vi "run.vi"(8 "error in (no error)":errorcluster, 11 "DL090130ExperimentController in":refnum<class "ExperimentControllerDL090130Interval.lvclass">=refnum) -> (0 "error out":errorcluster, 3 "DL090130ExperimentController out":refnum<class "ExperimentControllerDL090130Interval.lvclass">)   [LabVIEW 2010, in "ExperimentControllerDL090130Interval.lvclass"]
uses:
  ExperimentControllerDL090130Interval.lvclass
  common/classes/SpaceVector/SpaceVector/SpaceVector.lvclass
  Sweep/GenericSweep/GenericSweep/GenericSweep.lvclass
  schedule_entry_cluster.ctl
  internal_trigger_enum.ctl
  main/labview_source/controls/undock_button.ctl
  ExperimentControllerDL090130Interval.lvclass/ExperimentControllerDL090130Interval.ctl
  GenericExperimentController/GenericExperimentController/GenericExperimentController.lvclass
  common/classes/GenericToplevelComponent/GenericToplevelComponent/trigger_type_enum.ctl
  GenericExperimentController/GenericExperimentController/trigger_enum.ctl
  common/classes/ErrorController/ErrorController/class_data.vi
  common/classes/ErrorController/ErrorController/ErrorController.lvclass
panel:
  in  "button:undock":T1
  in  "Tab Control":enum32{"User", "Debug", "About"}(tab)
  in  "number of sweeps":i32=1
  in  "sweep period":dbl[unit]
  in  "current sweep":i32
  in  "configure sweep button":bool
  out "event str time-out":i32
  out "stop?":bool
  in  "scheduled triggers":T2[](array[typedef])
  out "any triggers scheduled?":bool
  out "time-out for next sweep":i32
  out "last time-out: trigger due?":bool
  out "last trigger":T2
  out "last trigger time":timestamp
  out "evnt loop error":errorcluster
  out "last trigger":T3
  out "event handling loop counter":i32=343
  # "Sweep period:  duration from the beginning of one sweep to the beginning of the next sweep.\nImportant: The sweep period has to be longer than the actual duration of the sweep (including possible saving)."
  # "ExperimentControllerDL090130Interval\n\nImplemented by:\nDominik Langer, University of Zurich, Switzerland"
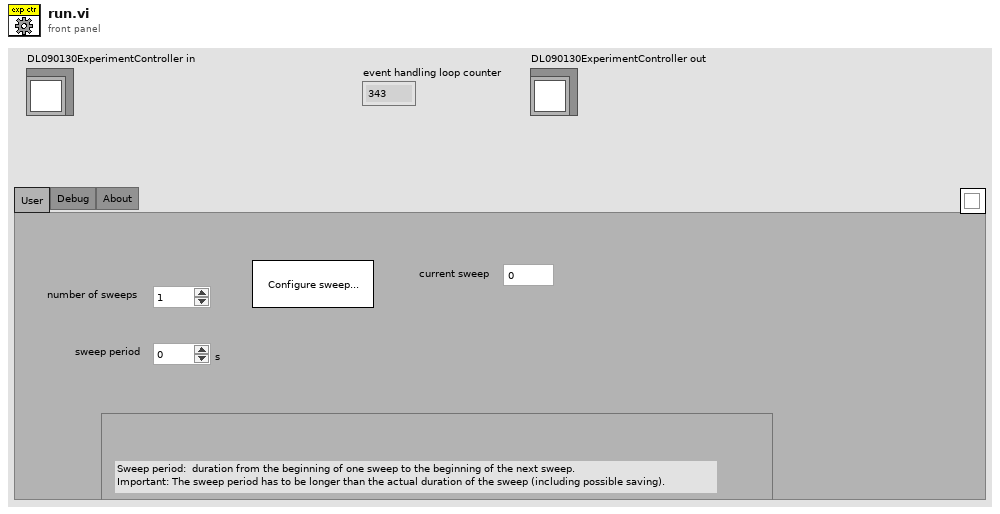
[diagram p1: front panel]
types:
  T1 = typedef "undock_button.ctl" = bool
  T2 = typedef "ExperimentControllerDL090130Interval.lvclass/schedule_entry_cluster.ctl" = cluster{"time":timestamp, "trigger":T3}
  T3 = typedef "ExperimentControllerDL090130Interval.lvclass/internal_trigger_enum.ctl" = enum16{"NULL", "initialise", "terminate", "start", "stop", "proceed", "prepare", "start sweep"}
  T4 = typedef "trigger_type_enum.ctl" = enum8{"external", "internal", "common"}
  T5 = typedef "GenericExperimentController.lvclass/trigger_enum.ctl" = enum16{"NULL", "proceed", "prepare"}
  T6 = typedef "top-level_component_type_enum.ctl" = enum16{"undefined", "ImagingMode", "ScanHead", "DAQ", "ImageAssembler", "Display", "DataCollection", "Analyser", "Stimulator", "ExperimentController", "Instrument", "Stage"}
  T7 = typedef "main_trigger_enum.ctl" = enum16{"NULL", "initialise", "terminate", "start", "stop", "change objective", "change experimentController", "change imagingMode", "save notebook", "started saving", "finished saving", "expCtr ready", "expCtr missing", "imgMd ready", "imgMd missing", "scanHd ready", "scanHd missing", "DAQ ready", "DAQ missing", "imgAsm ready", "imgAsm missing", "dataColl ready", "dataColl missing", "display ready", "display missing", "analysr ready", "analysr missing", "instrmnt ready", "instrmnt missing", "stimltr ready", "stimltr missing", "stage ready", "stage missing"}
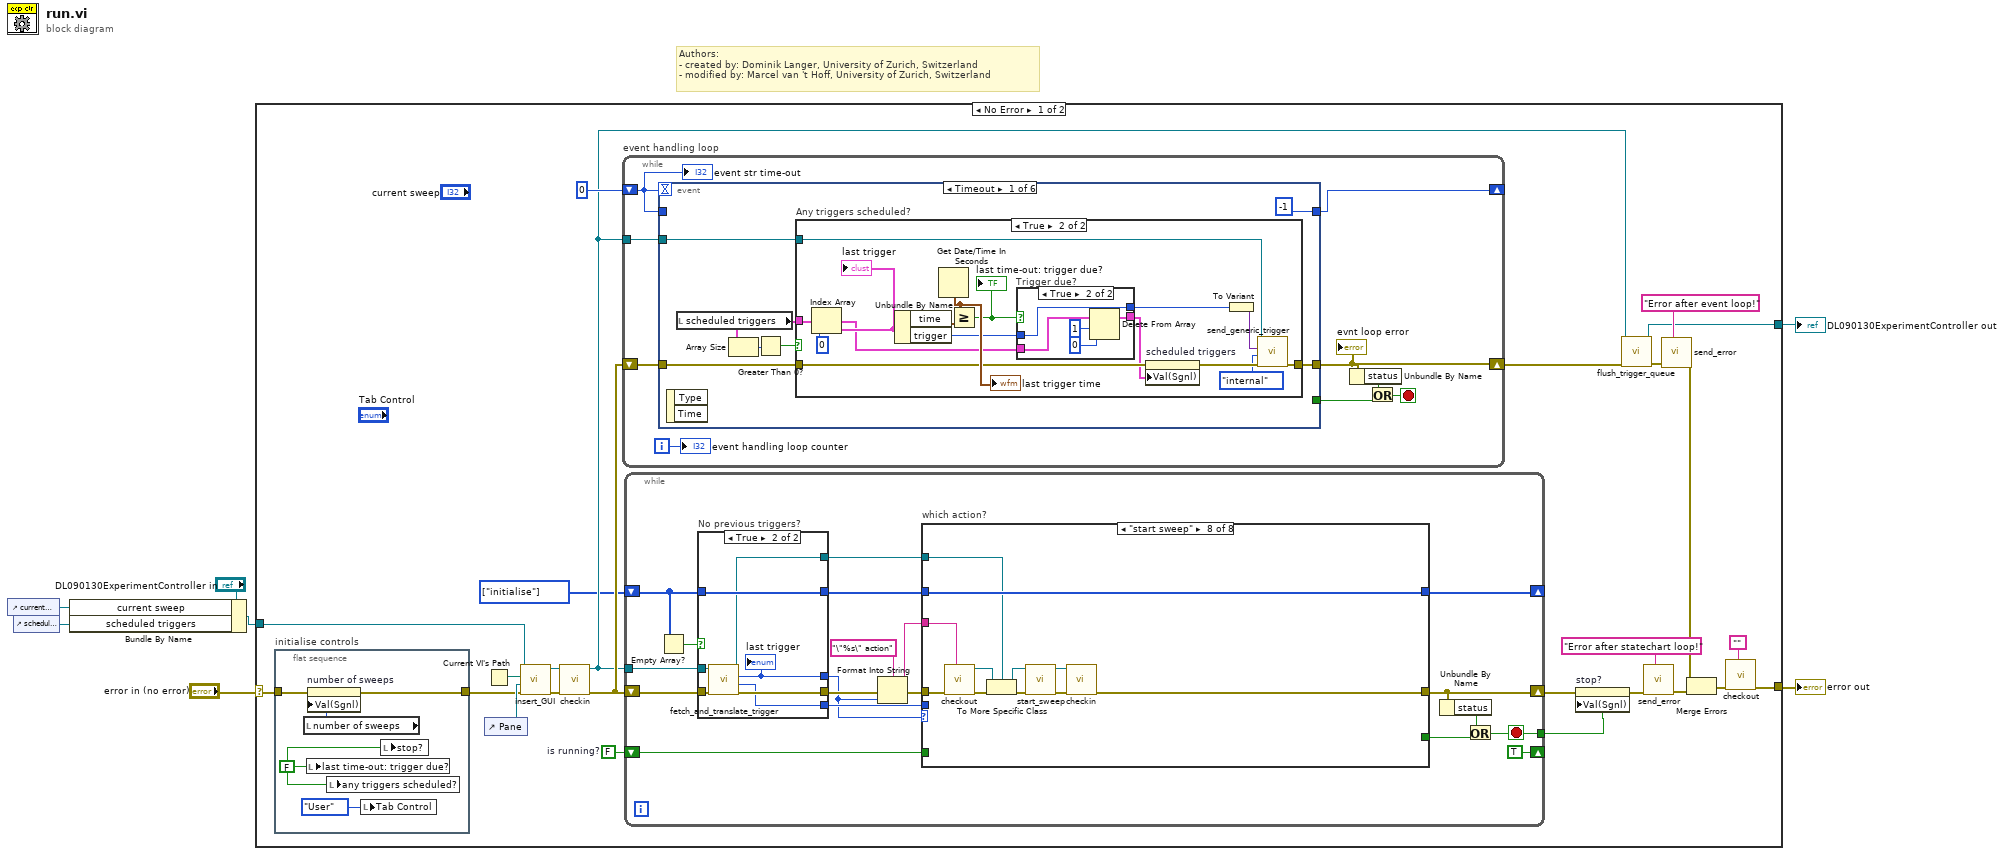
[diagram p0: block diagram]
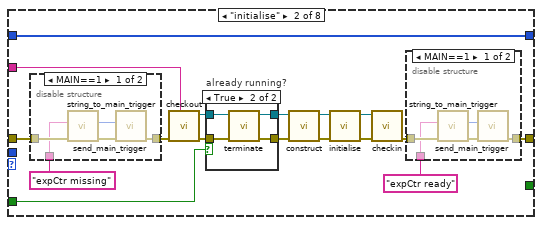
[diagram p3: hidden frame]
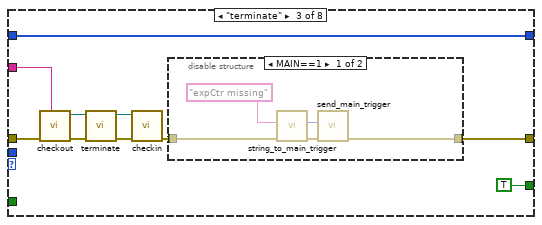
[diagram p7: hidden frame]
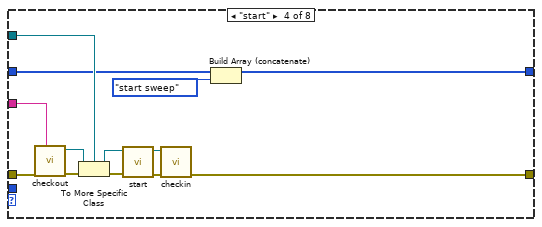
[diagram p9: hidden frame]
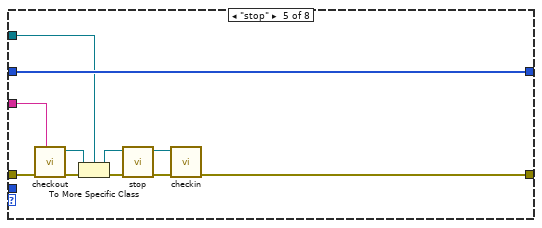
[diagram p10: hidden frame]
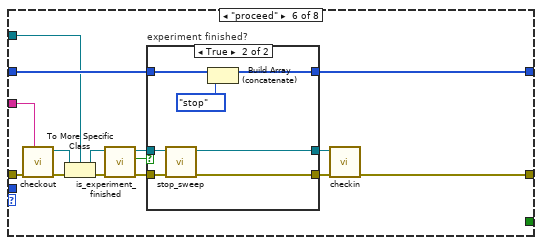
[diagram p11: hidden frame]
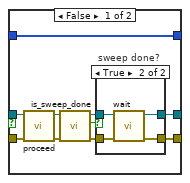
[diagram p12: hidden frame]
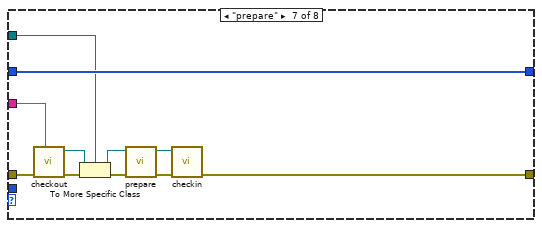
[diagram p14: hidden frame]
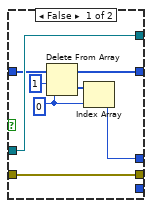
[diagram p15: hidden frame]
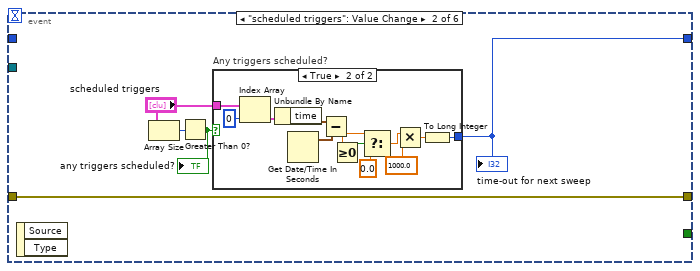
[diagram p18: hidden frame]
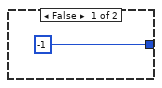
[diagram p19: hidden frame]
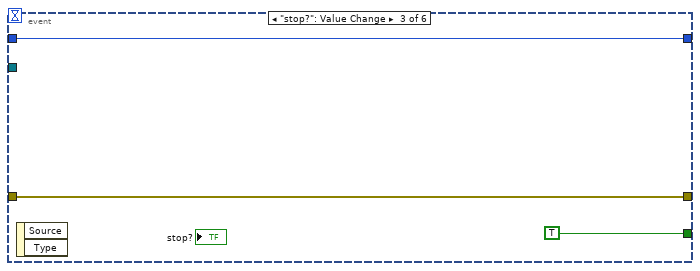
[diagram p20: hidden frame]
diagram:
  # "Authors: \n- created by: Dominik Langer, University of Zurich, Switzerland\n- modified by: Marcel van 't Hoff, University of Zurich, Switzerland"
  n1 = control-ref of="current sweep"() -> (w4:refnum<vi>)
  n2 = control-ref of="scheduled triggers"() -> (w1:refnum<vi>)
  n3 = Bundle By Name(cluster="DL090130ExperimentController in", "current sweep"=w4, "scheduled triggers"=w1) -> (w2:refnum<class "ExperimentControllerDL090130Interval.lvclass">)
  n4 = case shown="No Error" "error in (no error)" {
    selector: "error in (no error)" -> [w21 w306]
    tunnel: [w30 w306] -> w6
    tunnel: [w14 w305] -> w5
    tunnel: w2 -> [w20 w305]
    frame No Error {
      w10 = T3[] [enum."initialise"] items=["NULL", "initialise", "terminate", "start", "stop", "proceed", "prepare", "start sweep"]
      w11 = FALSE  # is running?
      n5 = flat-sequence "initialise controls" {
        tunnel: [w207] -> w17
        tunnel: w21 -> [w206]
        frame #0 {
          w205 = FALSE ("stop?")
          n6 = local read "number of sweeps"() -> (w208:i32)
          n7 = local write "last time-out: trigger due?"(w205) -> ()
          n8 = property on="number of sweeps" class="DigNum (strict)"(error in=w206, "Val(Sgnl)"=w208) -> (error out=w207:errorcluster)  [unwired: 1 in, 1 out]
          n9 = local write "any triggers scheduled?"(w205) -> ()
          n10 = local write "Tab Control"(enum32{"User", "Debug", "About"}."User" ("Tab Control")) -> ()
          n11 = local write "stop?"(w205) -> ()
        }
      }
      n12 = Current VI's Path() -> (path=w28:path)
      n13 = control-ref of="Pane"() -> (w27:refnum<vi>)
      n14 = call-dynamic "insert_GUI.vi"("error in (no error)"=w17, "Pane"=w27, "VI path"=w28, "GenericComponent in"=w20) -> ("error out"=w18:errorcluster, "GenericComponent out"=w19:refnum<class "ExperimentControllerDL090130Interval.lvclass">)  [unwired: 6 in]
      n15 = call-dynamic "checkin.vi"("error in (no error)"=w18, "GenericExperimentController in"=w19) -> ("error out"=w13:errorcluster, "GenericExperimentController out"=w12:refnum<class "ExperimentControllerDL090130Interval.lvclass">)  [unwired: 8 in]
      n16 = while "event handling loop" {
        shift-right: [w212] -> w16
        shift-left: w13 -> [w217]
        shift-right: [w215] -> _
        shift-left: 0 ("statechart creation time") -> [w216]
        tunnel: w12 -> [w213]
        i -> [w214]
        stop <- w209 stop-if-true
        n17 = event shown="[0] Timeout" {
          selector: _ -> [_ _ _ _ _ _]
          dyn-events: _ -> [_ _ _ _ _ _]
          timeout: w216 -> [_ _ _ _ _ _]
          tunnel: w217 -> [w220 w251 w267 w282 w297 w302]
          tunnel: [w219 w251 w267 w281 w283 w301] -> w212
          tunnel: [-1 ("statechart creation time") w247 w266 w274 w298 w304] -> w215
          tunnel: w216 -> [_ _ w266 w274 w298 w304]
          tunnel: [_ _ TRUE _ _ _] -> w211
          tunnel: w213 -> [w218 _ _ _ w287 w303]
          event Timeout {
            n18 = event-data() -> ()  [unwired: 3 out]
            n19 = local read "scheduled triggers"() -> (w221:T2[])
            n20 = Array Size(array=w221) -> (size(s)=w223:i32)
            n21 = Greater Than 0?(x=w223) -> (x > 0?=w222:bool)
            n22 = case "Any triggers scheduled?" shown="True" w222 {
              tunnel: w221 -> [_ w235]
              tunnel: w220 -> [w225 w233]
              tunnel: [w225 w227] -> w219
              tunnel: w218 -> [_ w231]
              frame False {
              }
              frame True {
                n23 = Index Array(array=w235, index=0) -> (element=w238:T2)
                "last trigger" <- w238
                n24 = Unbundle By Name(w238) -> ("time"=w240:timestamp, "trigger"=w234:T3)
                n25 = Get Date/Time In Seconds() -> (seconds since 1Jan1904=w239:timestamp)
                "last trigger time" <- w239
                n26 = Greater Or Equal?(x=w239, y=w240) -> (x >= y?=w236:bool)
                "last time-out: trigger due?" <- w236
                n27 = case "Trigger due?" shown="True" w236 {
                  tunnel: w235 -> [w241 w244]
                  tunnel: w234 -> [_ w243]
                  tunnel: [_ w243] -> w230
                  tunnel: [w241 w242] -> w232
                  frame False {
                  }
                  frame True {
                    n28 = Delete From Array(array=w244, length=1, index=0) -> (array with subset deleted=w242:T2[])  [unwired: 1 out]
                  }
                }
                n29 = property on="scheduled triggers" class="Arr (strict)"(error in=w233, "Val(Sgnl)"=w232) -> (error out=w228:errorcluster)  [unwired: 1 in, 1 out]
                n30 = To Variant(anything=w230) -> (Variant=w229:variant)
                n31 = call-dynamic "send_generic_trigger.vi"("error in (no error)"=w228, "trigger type"=trigger_type_enum."internal", "trigger variant"=w229, "GenericToplevelComponent in"=w231) -> ("error out"=w227:errorcluster)  [unwired: 4 in, 3 out]
              }
            }
          }
          event "scheduled triggers": Value Change {
            n32 = event-data() -> ()  [unwired: 3 out]
            n33 = Array Size(array="scheduled triggers") -> (size(s)=w250:i32)
            n34 = Greater Than 0?(x=w250) -> (x > 0?=w248:bool)
            "any triggers scheduled?" <- w248
            n35 = case "Any triggers scheduled?" shown="True" w248 {
              tunnel: [-1 w259] -> w247
              tunnel: "scheduled triggers" -> [_ w260]
              frame False {
              }
              frame True {
                n36 = Index Array(array=w260, index=0) -> (element=w263:T2)
                n37 = Unbundle By Name(w263) -> ("time"=w262:timestamp)
                n38 = Get Date/Time In Seconds() -> (seconds since 1Jan1904=w261:timestamp)
                n39 = Subtract(x=w262, y=w261) -> (x-y=w255:dbl)
                n40 = Greater Or Equal To 0?(x=w255) -> (x >= 0?=w256:bool)
                n41 = Select(t=w255, s=w256, f=0.0) -> (s? t:f=w254:dbl)
                n42 = Multiply(x=w254, y=1000.0) -> (x*y=w258:dbl)
                n43 = To Long Integer(number=w258) -> (32bit integer=w259:i32)
              }
            }
            "time-out for next sweep" <- w247
          }
          event "stop?": Value Change {
            n44 = event-data() -> ()  [unwired: 3 out]
          }
          event "number of sweeps", "sweep period": Value Change {
            n45 = event-data() -> ()  [unwired: 2 out]
            n46 = call "checkout.vi"("locked by?"="number of sweeps/sweep period: value change" ("string"), "error in (no error)"=w282) -> ("error out"=w279:errorcluster, "GenericExperimentController out"=w278:refnum<class "GenericExperimentController.lvclass">)  [unwired: 1 in, 7 out]
            n47 = To More Specific Class(target class=refnum<class "ExperimentControllerDL090130Interval.lvclass"> refnum ("DL090130ExperimentController.lvclass"), reference=w278, error in=w279) -> (specific class reference=w275:refnum<class "ExperimentControllerDL090130Interval.lvclass">, error out=w277:errorcluster)
            n48 = call "set_number_of_sweeps.vi"("error in (no error)"=w277, "number of sweeps"="number of sweeps", "DL090130ExperimentController.lvclass in"=w275) -> ("error out"=w273:errorcluster, "DL090130ExperimentController.lvclass out"=w271:refnum<class "ExperimentControllerDL090130Interval.lvclass">)  [unwired: 7 out]
            n49 = call "set_sweep_period.vi"("error in (no error)"=w273, "sweep period"="sweep period", "DL090130ExperimentController.lvclass in"=w271) -> ("error out"=w269:errorcluster, "DL090130ExperimentController.lvclass out"=w268:refnum<class "ExperimentControllerDL090130Interval.lvclass">)  [unwired: 7 out]
            n50 = call-dynamic "checkin.vi"("error in (no error)"=w269, "GenericExperimentController in"=w268) -> ("error out"=w281:errorcluster)  [unwired: 8 in, 1 out]
          }
          event "configure sweep button": Value Change {
            n51 = event-data() -> ()  [unwired: 2 out]
            n52 = call "checkout.vi"("locked by?"="\"configure sweep button\": value change", "error in (no error)"=w297) -> ("error out"=w295:errorcluster, "GenericExperimentController out"=w294:refnum<class "GenericExperimentController.lvclass">)  [unwired: 8 in]
            n53 = To More Specific Class(target class=w287, reference=w294, error in=w295) -> (specific class reference=w293:refnum<class "ExperimentControllerDL090130Interval.lvclass">, error out=w291:errorcluster)
            n54 = Unbundle By Name(w293) -> ("sweep"=w289:refnum<class "GenericSweep.lvclass">)
            n55 = call-dynamic "configure.vi"("error in (no error)"=w291, "GenericPlugin in"=w289) -> ("error out"=w290:errorcluster, "GenericPlugin out"=w288:refnum<class "GenericSweep.lvclass">)  [unwired: 8 in]
            n56 = Bundle By Name(cluster=w293, "sweep"=w288) -> (w292:refnum<class "ExperimentControllerDL090130Interval.lvclass">)
            n57 = call-dynamic "checkin.vi"("error in (no error)"=w290, "GenericExperimentController in"=w292) -> ("error out"=w286:errorcluster, "GenericExperimentController out"=w284:refnum<class "ExperimentControllerDL090130Interval.lvclass">)  [unwired: 8 in]
            n58 = call-dynamic "send_trigger.vi"("error in (no error)"=w286, "trigger"=trigger_enum."proceed", "GenericExperiment in"=w284) -> ("error out"=w283:errorcluster)  [unwired: 7 in, 1 out]
          }
          event Value Change {
            n59 = event-data() -> ()  [unwired: 2 out]
            n60 = Current VI's Path() -> (path=w299:path)
            n61 = call-dynamic "undock.vi"("error in (no error)"=w302, "undock?"="button:undock", "VI path"=w299, "GenericComponent in"=w303) -> ("error out"=w301:errorcluster)  [unwired: 6 in, 1 out]
          }
        }
        "evnt loop error" <- w212
        n62 = Unbundle By Name(w212) -> ("status"=w210:bool)
        n63 = Or(x=w210, y=w211) -> (x .or. y?=w209:bool)
        "event handling loop counter" <- w214
        "event str time-out" <- w216
      }
      n64 = while {
        shift-right: [w37] -> w8
        shift-left: w13 -> [w51]
        shift-right: [w43] -> _
        shift-left: w10 -> [w48]
        shift-right: [TRUE ("is running?")] -> _
        shift-left: w11 -> [w40]
        tunnel: w12 -> [w50]
        tunnel: [w34] -> w9
        stop <- w34 stop-if-true
        n65 = Empty Array?(array=w48) -> (empty?=w49:bool)
        n66 = case "No previous triggers?" shown="True" w49 {
          tunnel: w50 -> [w196 w201]
          tunnel: w51 -> [w194 w202]
          tunnel: [w196 w200] -> w44
          tunnel: [w192 w198] -> w33
          tunnel: [_ w197] -> w38
          tunnel: [w194 w199] -> w46
          tunnel: w48 -> [w195 w203]
          tunnel: [w191 w203] -> w42
          frame False {
            w189 = 0 ("index")
            n67 = Delete From Array(array=w195, length=1, index=w189) -> (deleted portion=w193:T3[], array with subset deleted=w191:T3[])
            n68 = Index Array(array=w193, index=w189) -> (element=w192:T3)
          }
          frame True {
            n69 = call-dynamic "fetch_and_translate_trigger.vi"("error in (no error)"=w202, "ExperimentControllerDL090130Interval in"=w201) -> ("error out"=w199:errorcluster, "sender TLC type"=w197:T6, "trigger"=w198:T3, "ExperimentControllerDL090130Interval out"=w200:refnum<class "ExperimentControllerDL090130Interval.lvclass">)  [unwired: 6 in]
            "last trigger" <- w198
          }
        }
        n70 = Format Into String(format string="\"%s\" action", error in=w46, w33) -> (resulting string=w41:string, error out=w45:errorcluster)  [unwired: 1 in]
        n71 = case "which action?" shown="\"start sweep\"" w33 {
          tunnel: [w52 w61 w89 w112 w125 w133 w167 w178] -> w37
          tunnel: w45 -> [w52 w69 w94 w113 w122 w138 w170 w184]
          tunnel: w44 -> [_ _ _ w110 w123 w137 w168 w183]
          tunnel: [w53 w70 w98 w106 w128 w141 w177 w188] -> w43
          tunnel: w42 -> [w53 w70 w98 w107 w128 w142 w177 w188]
          tunnel: w41 -> [_ w65 w93 w111 w124 w139 w169 w185]
          tunnel: w40 -> [_ w60 _ _ _ _ _ _]
          tunnel: w38 -> [_ _ _ _ _ _ _ _]
          tunnel: [_ _ TRUE _ _ _ _ _] -> w36
          frame "NULL", Default {
          }
          frame "initialise" {
            n72 = disable-structure shown="MAIN==1" {
              disable-tunnel: w69 -> [w85 w88]
              disable-tunnel: [w87 w88] -> w66
              disable-tunnel: "expCtr missing" -> [w83 _]
              frame condition #0 {
                n73 = call "string_to_main_trigger.vi"("error in (no error)"=w85, "trigger string"=w83) -> ("error out"=w84:errorcluster, "main trigger"=w86:T7)  [unwired: 8 in]
                n74 = call "send_main_trigger.vi"("error in (no error)"=w84, "trigger"=w86) -> ("error out"=w87:errorcluster)  [unwired: 9 in]
              }
              frame condition #1 (active) {
              }
            }
            n75 = call "checkout.vi"("locked by?"=w65, "error in (no error)"=w66) -> ("error out"=w57:errorcluster, "GenericExperimentController out"=w59:refnum<class "GenericExperimentController.lvclass">)  [unwired: 1 in, 7 out]
            n76 = case "already running?" shown="True" w60 {
              tunnel: w59 -> [w72 w76]
              tunnel: [w72 w75] -> w58
              tunnel: w57 -> [w71 w74]
              tunnel: [w71 w73] -> w56
              frame False {
              }
              frame True {
                n77 = call-dynamic "terminate.vi"("error in (no error)"=w74, "GenericPlugin in"=w76) -> ("error out"=w73:errorcluster, "GenericPlugin out"=w75:refnum<class "GenericExperimentController.lvclass">)  [unwired: 8 in]
              }
            }
            n78 = call-dynamic "construct.vi"("error in (no error)"=w56, "GenericPlugin in"=w58) -> ("error out"=w68:errorcluster, "GenericPlugin out"=w63:refnum<class "GenericExperimentController.lvclass">)  [unwired: 2 in, 6 out]
            n79 = call-dynamic "initialise.vi"("error in (no error)"=w68, "GenericPlugin in"=w63) -> ("error out"=w67:errorcluster, "GenericPlugin out"=w64:refnum<class "GenericExperimentController.lvclass">)  [unwired: 8 out]
            n80 = call-dynamic "checkin.vi"("error in (no error)"=w67, "GenericExperimentController in"=w64) -> ("error out"=w62:errorcluster)  [unwired: 8 in, 1 out]
            n81 = disable-structure shown="MAIN==1" {
              disable-tunnel: w62 -> [w80 w82]
              disable-tunnel: [w81 w82] -> w61
              disable-tunnel: "expCtr ready" -> [w77 _]
              frame condition #0 {
                n82 = call "string_to_main_trigger.vi"("error in (no error)"=w80, "trigger string"=w77) -> ("error out"=w79:errorcluster, "main trigger"=w78:T7)  [unwired: 8 in]
                n83 = call "send_main_trigger.vi"("error in (no error)"=w79, "trigger"=w78) -> ("error out"=w81:errorcluster)  [unwired: 9 in]
              }
              frame condition #1 (active) {
              }
            }
          }
          frame "terminate" {
            n84 = call "checkout.vi"("locked by?"=w93, "error in (no error)"=w94) -> ("error out"=w95:errorcluster, "GenericExperimentController out"=w91:refnum<class "GenericExperimentController.lvclass">)  [unwired: 1 in, 7 out]
            n85 = call-dynamic "terminate.vi"("error in (no error)"=w95, "GenericPlugin in"=w91) -> ("error out"=w96:errorcluster, "GenericPlugin out"=w92:refnum<class "GenericExperimentController.lvclass">)  [unwired: 8 out]
            n86 = call-dynamic "checkin.vi"("error in (no error)"=w96, "GenericExperimentController in"=w92) -> ("error out"=w90:errorcluster)  [unwired: 8 in, 1 out]
            n87 = disable-structure shown="MAIN==1" {
              disable-tunnel: w90 -> [w100 w104]
              disable-tunnel: [w103 w104] -> w89
              frame condition #0 {
                n88 = call "string_to_main_trigger.vi"("error in (no error)"=w100, "trigger string"="expCtr missing") -> ("error out"=w99:errorcluster, "main trigger"=w101:T7)  [unwired: 8 in]
                n89 = call "send_main_trigger.vi"("error in (no error)"=w99, "trigger"=w101) -> ("error out"=w103:errorcluster)  [unwired: 9 in]
              }
              frame condition #1 (active) {
              }
            }
          }
          frame "start" {
            n90 = call "checkout.vi"("locked by?"=w111, "error in (no error)"=w113) -> ("error out"=w114:errorcluster, "GenericExperimentController out"=w117:refnum<class "GenericExperimentController.lvclass">)  [unwired: 8 in]
            n91 = To More Specific Class(target class=w110, reference=w117, error in=w114) -> (specific class reference=w116:refnum<class "ExperimentControllerDL090130Interval.lvclass">, error out=w115:errorcluster)
            n92 = call-dynamic "start.vi"("error in (no error)"=w115, "ExperimentControllerDL090130Interval in"=w116) -> ("error out"=w108:errorcluster, "ExperimentControllerDL090130Interval out"=w109:refnum<class "ExperimentControllerDL090130Interval.lvclass">)  [unwired: 8 in]
            n93 = call-dynamic "checkin.vi"("error in (no error)"=w108, "GenericExperimentController in"=w109) -> ("error out"=w112:errorcluster)  [unwired: 8 in, 1 out]
            n94 = Build Array (concatenate)(w107, internal_trigger_enum."start sweep" ("internal trigger enum")) -> (w106:T3[])
          }
          frame "stop" {
            n95 = call "checkout.vi"("locked by?"=w124, "error in (no error)"=w122) -> ("error out"=w126:errorcluster, "GenericExperimentController out"=w127:refnum<class "GenericExperimentController.lvclass">)  [unwired: 8 in]
            n96 = To More Specific Class(target class=w123, reference=w127, error in=w126) -> (specific class reference=w119:refnum<class "ExperimentControllerDL090130Interval.lvclass">, error out=w118:errorcluster)
            n97 = call-dynamic "stop.vi"("error in (no error)"=w118, "ExperimentControllerDL090130Interval in"=w119) -> ("error out"=w121:errorcluster, "ExperimentControllerDL090130Interval out"=w120:refnum<class "ExperimentControllerDL090130Interval.lvclass">)  [unwired: 8 in]
            n98 = call-dynamic "checkin.vi"("error in (no error)"=w121, "GenericExperimentController in"=w120) -> ("error out"=w125:errorcluster)  [unwired: 8 in, 1 out]
          }
          frame "proceed" {
            n99 = call "checkout.vi"("locked by?"=w139, "error in (no error)"=w138) -> ("error out"=w140:errorcluster, "GenericExperimentController out"=w136:refnum<class "GenericExperimentController.lvclass">)  [unwired: 8 in]
            n100 = To More Specific Class(target class=w137, reference=w136, error in=w140) -> (specific class reference=w130:refnum<class "ExperimentControllerDL090130Interval.lvclass">, error out=w129:errorcluster)
            n101 = call-dynamic "is_experiment_finished.vi"("error in (no error)"=w129, "DL090130ExperimentController in"=w130) -> ("error out"=w134:errorcluster, "is finished?"=w143:bool, "DL090130ExperimentController out"=w135:refnum<class "ExperimentControllerDL090130Interval.lvclass">)  [unwired: 7 out]
            n102 = case "experiment finished?" shown="True" w143 {
              tunnel: [w151 w161] -> w132
              tunnel: w135 -> [w147 w162]
              tunnel: w134 -> [w146 w163]
              tunnel: [w148 w165] -> w141
              tunnel: w142 -> [w148 w166]
              tunnel: [w149 w160] -> w131
              frame False {
                n103 = call-dynamic "proceed.vi"("error in (no error)"=w146, "ExperimentControllerDL090130Interval in"=w147) -> ("error out"=w145:errorcluster, "ExperimentControllerDL090130Interval out"=w144:refnum<class "ExperimentControllerDL090130Interval.lvclass">)  [unwired: 8 in]
                n104 = call-dynamic "is_sweep_done.vi"("error in (no error)"=w145, "ExperimentControllerDL090130Interval in"=w144) -> ("error out"=w153:errorcluster, "sweep done?"=w152:bool, "ExperimentControllerDL090130Interval out"=w150:refnum<class "ExperimentControllerDL090130Interval.lvclass">)  [unwired: 7 in]
                n105 = case "sweep done?" shown="True" w152 {
                  tunnel: w153 -> [w155 w157]
                  tunnel: [w155 w156] -> w151
                  tunnel: w150 -> [w154 w159]
                  tunnel: [w154 w158] -> w149
                  frame False {
                  }
                  frame True {
                    n106 = call-dynamic "wait.vi"("error in (no error)"=w157, "DL090130ExperimentController in"=w159) -> ("error out"=w156:errorcluster, "DL090130ExperimentController out"=w158:refnum<class "ExperimentControllerDL090130Interval.lvclass">)  [unwired: 8 out]
                  }
                }
              }
              frame True {
                n107 = call-dynamic "stop_sweep.vi"("error in (no error)"=w163, "DL090130ExperimentController in"=w162) -> ("error out"=w161:errorcluster, "DL090130ExperimentController out"=w160:refnum<class "ExperimentControllerDL090130Interval.lvclass">)  [unwired: 8 in]
                n108 = Build Array (concatenate)(w166, internal_trigger_enum."stop" ("internal trigger enum")) -> (w165:T3[])
              }
            }
            n109 = call-dynamic "checkin.vi"("error in (no error)"=w132, "GenericExperimentController in"=w131) -> ("error out"=w133:errorcluster)  [unwired: 8 in, 1 out]
          }
          frame "prepare" {
            n110 = call "checkout.vi"("locked by?"=w169, "error in (no error)"=w170) -> ("error out"=w171:errorcluster, "GenericExperimentController out"=w176:refnum<class "GenericExperimentController.lvclass">)  [unwired: 8 in]
            n111 = To More Specific Class(target class=w168, reference=w176, error in=w171) -> (specific class reference=w175:refnum<class "ExperimentControllerDL090130Interval.lvclass">, error out=w172:errorcluster)
            n112 = call-dynamic "prepare.vi"("error in (no error)"=w172, "ExperimentControllerDL090130Interval in"=w175) -> ("error out"=w173:errorcluster, "ExperimentControllerDL090130Interval out"=w174:refnum<class "ExperimentControllerDL090130Interval.lvclass">)  [unwired: 8 in]
            n113 = call-dynamic "checkin.vi"("error in (no error)"=w173, "GenericExperimentController in"=w174) -> ("error out"=w167:errorcluster)  [unwired: 8 in, 1 out]
          }
          frame "start sweep" {
            n114 = call "checkout.vi"("locked by?"=w185, "error in (no error)"=w184) -> ("error out"=w186:errorcluster, "GenericExperimentController out"=w187:refnum<class "GenericExperimentController.lvclass">)  [unwired: 8 in]
            n115 = To More Specific Class(target class=w183, reference=w187, error in=w186) -> (specific class reference=w181:refnum<class "ExperimentControllerDL090130Interval.lvclass">, error out=w182:errorcluster)
            n116 = call-dynamic "start_sweep.vi"("error in (no error)"=w182, "DL090130ExperimentController in"=w181) -> ("error out"=w180:errorcluster, "DL090130ExperimentController out"=w179:refnum<class "ExperimentControllerDL090130Interval.lvclass">)  [unwired: 8 out]
            n117 = call-dynamic "checkin.vi"("error in (no error)"=w180, "GenericExperimentController in"=w179) -> ("error out"=w178:errorcluster)  [unwired: 8 in, 1 out]
          }
        }
        n118 = Unbundle By Name(w37) -> ("status"=w35:bool)
        n119 = Or(x=w35, y=w36) -> (x .or. y?=w34:bool)
      }
      n120 = property on="stop?" class="Bool (strict)"(error in=w8, "Val(Sgnl)"=w9) -> (error out=w26:errorcluster)  [unwired: 1 in, 1 out]
      n121 = call-dynamic "flush_trigger_queue.vi"("error in (no error)"=w16, "GenericToplevelComponent in"=w12) -> ("error out"=w15:errorcluster, "GenericToplevelComponent out"=w14:refnum<class "ExperimentControllerDL090130Interval.lvclass">)  [unwired: 8 in]
      n122 = call "send_error.vi"("additional message"="Error after statechart loop!", "error in (no error)"=w26) -> ("error out"=w25:errorcluster)  [unwired: 9 in]
      n123 = call "send_error.vi"("additional message"="Error after event loop!", "error in (no error)"=w15) -> ("error out"=w24:errorcluster)  [unwired: 9 in]
      n124 = Merge Errors(w24, w25) -> (w31:errorcluster)
      n125 = call "checkout.vi"("locked by?"="", "error in (no error)"=w31) -> ("error out"=w30:errorcluster)  [unwired: 1 in, 8 out]
    }
    frame Error {
    }
  }
  "error out" <- w6
  "DL090130ExperimentController out" <- w5
